vi "orion.vi"(9 "freq":dbl, 10 "csi":cdb[](array[numeric]), 11 "csi num":u32) -> (0 "error out":errorcluster, 1 "max":dbl, 2 "spectrum":cluster{dbl[], dbl[]}(graph), 3 "CSI abs":dbl[][](array[numeric]))   [LabVIEW 2020]
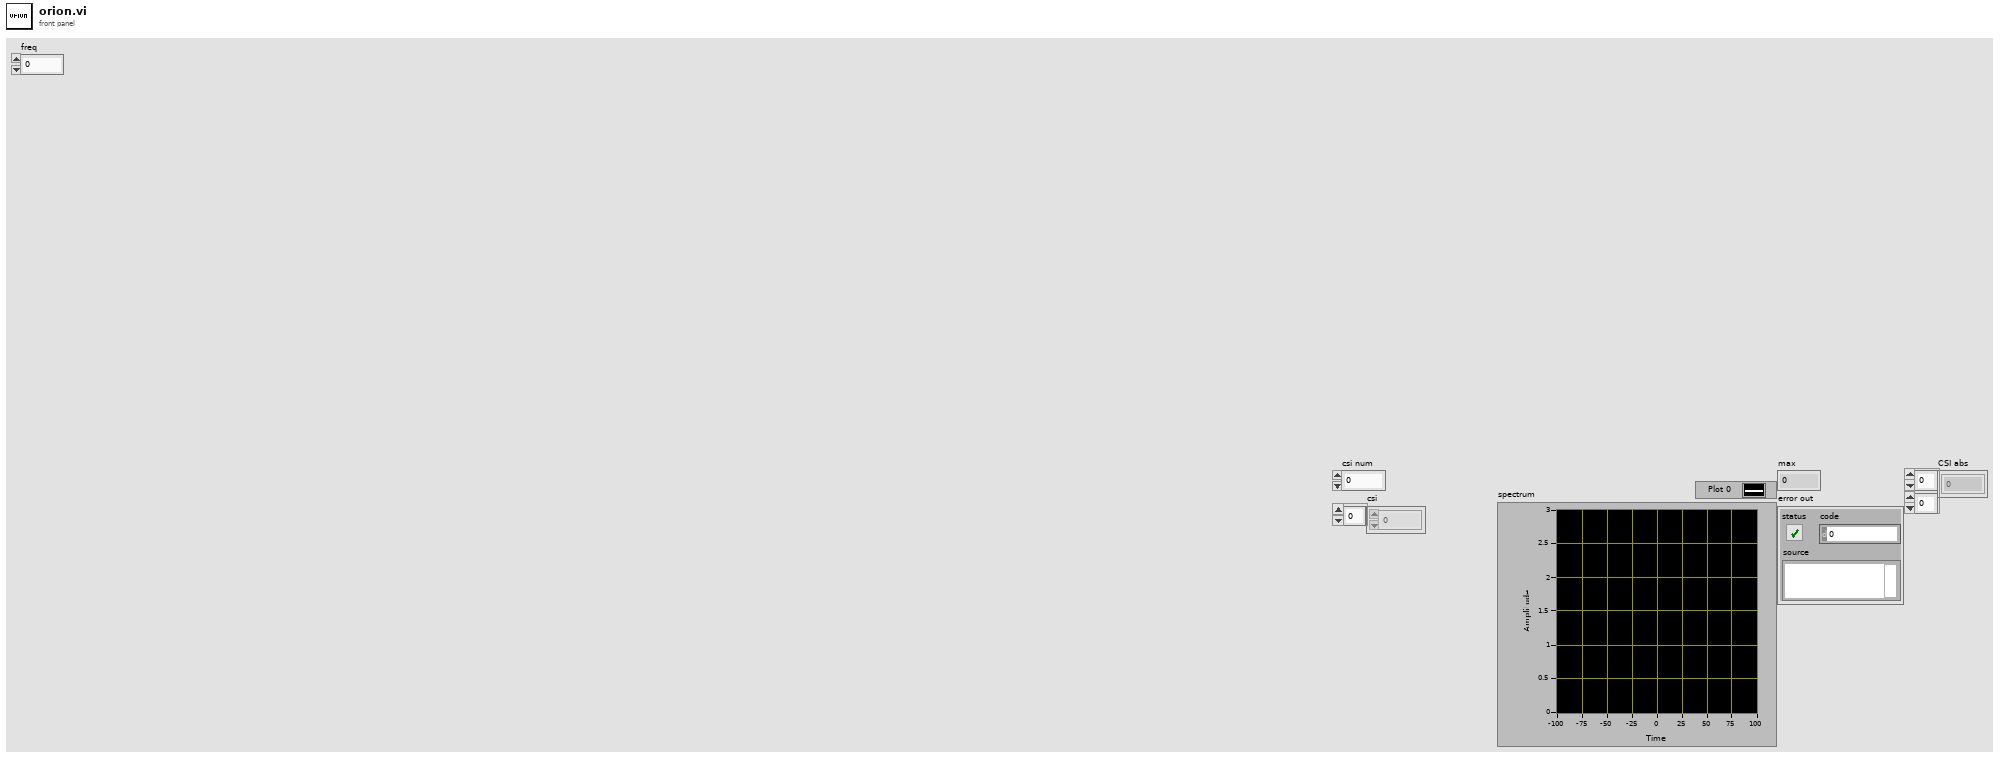
[diagram p1: front panel]
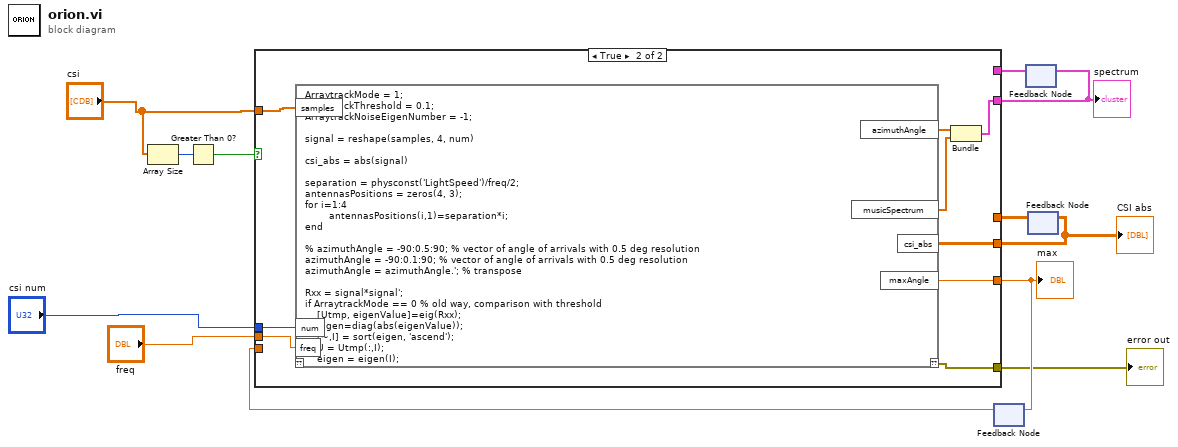
[diagram p0: block diagram]
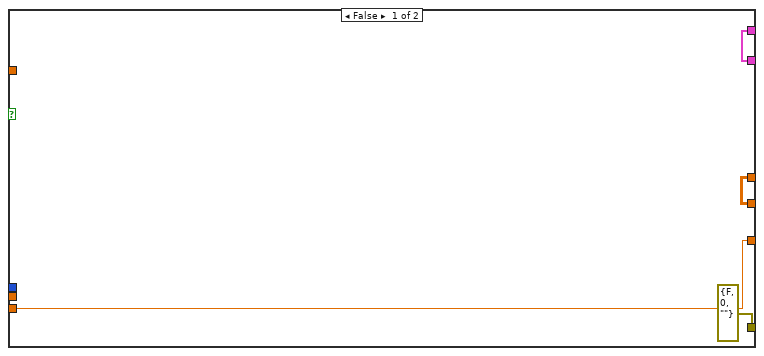
[diagram p2: hidden frame]
diagram:
  n1 = Array Size(array="csi") -> (size(s)=w6:i32)
  n2 = Greater Than 0?(x=w6) -> (x > 0?=w5:bool)
  n3 = feedback #1() -> (w10:dbl)  [unwired: 1 in]
  n4 = feedback #2() -> (w1:cluster{dbl[], dbl[]})  [unwired: 1 in]
  n5 = feedback #3() -> (w2:dbl[][])  [unwired: 1 in]
  n6 = case shown="True" w5 {
    tunnel: "freq" -> [_ w25]
    tunnel: [w13 w22] -> w12
    tunnel: [w16 w21] -> w11
    tunnel: w10 -> [w16 _]
    tunnel: "csi" -> [_ w18]
    tunnel: "csi num" -> [_ w20]
    tunnel: [errorcluster {"status"=FALSE, "code"=0, "source"=""} ("error IO") w19] -> w4
    tunnel: [w14 w17] -> w3
    tunnel: w2 -> [w14 _]
    tunnel: w1 -> [w13 _]
    frame False {
    }
    frame True {
      n7 = script code="ArraytrackMode = 1;\nArraytrackThreshold = 0.1;\nArraytrackNoiseEigenNumber = -1;\n\nsignal = reshape(samples, 4, num)\n\ncsi_abs = abs(signal)\n\nseparation = physconst('LightSpeed')/freq/2;\nantennasPositions = zeros(4, 3);\nfor i=1:4\n        antennasPositions(i,1)=separation*i;\nend\n\n% azimuthAngle = -90:0.5:90; % vector of angle of arrivals with 0.5 deg resolution\nazimuthAngle = -90:0.1:90; % vector of angle of arrivals with 0.5 deg resolution\nazimuthAngle = azimuthAngle.'; % transpose\n\nRxx = signal*signal';\nif ArraytrackMode == 0 % old way, comparison with threshold\n    [Utmp, eigenValue]=eig(Rxx);\n    eigen=diag(abs(eigenValue));\n    [~,I] = sort(eigen, 'ascend');\n    U = Utmp(:,I);\n    eigen = eigen(I);\n    \n    N = 0;\n    for i=1:size(antennasPositions,1)\n        if eigen(i) < ArraytrackThreshold\n            N = i;\n        end\n    end\n    \n    if N == 0\n        N = 1;\n    end\n    \n    En = U(:,1:N);\n    \n    if N == 0\n        error('Arraytrack: sources not found')\n    end\nelseif ArraytrackMode == 1\n    [Utmp,eigenValue] = eig(Rxx);\n    eigen=diag(abs(eigenValue));\n    [~,I] = sort(eigen, 'ascend');\n    U = Utmp(:,I);\n    eigen = eigen(I);\n    \n    N = ArraytrackNoiseEigenNumber;\n    if N < 0\n        N = length(eigen)+N;\n    end\n    En = U(:,1:N);\nend\n\nelevationAngle = zeros(size(azimuthAngle)); % vector of zeros with the same size as az\nsteeringVectors = steeringVectorsCreate(antennasPositions, [azimuthAngle + 90,elevationAngle], freq);\nmusicSpectrum=zeros(1,length(azimuthAngle));\nfor i=1:length(azimuthAngle)\n    musicSpectrum(i)=-10*log10(abs(steeringVectors(:,i)'*(En*En')*steeringVectors(:,i)));\nend\n%musicSpectrum = musicSpectrum.';\nmusicSpectrum = musicSpectrum - min(musicSpectrum);\n\n[~, ind] = max(musicSpectrum);\nif length(azimuthAngle) > 0\n    maxAngle = azimuthAngle(ind);\nend\n\nazimuthAngle = azimuthAngle.'; % transpose" ("Script Node")("samples"=w18, "num"=w20, "freq"=w25) -> ("??"=w19:errorcluster, "musicSpectrum"=w23:dbl[], "azimuthAngle"=w24:dbl[], "maxAngle"=w21:dbl, "csi_abs"=w17:dbl[][])  [unwired: 1 in]
      n8 = Bundle(w24, w23) -> (w22:cluster{dbl[], dbl[]})  [unwired: 1 in]
    }
  }
  "spectrum" <- w12
  "max" <- w11
  "error out" <- w4
  "CSI abs" <- w3
  n9 = feedback-in #1(w11) -> ()
  n10 = feedback-in #2(w12) -> ()
  n11 = feedback-in #3(w3) -> ()
